vi "HK Channel Read Formatted Value.vi"(8 "error in (no error)":errorcluster, 10 "Name":string, 11 "HK Channel in":refnum<class "HK Table.lvclass">) -> (0 "error out":errorcluster, 1 "Units":string, 2 "Value Formatted":string, 3 "HK Channel out":refnum<class "HK Table.lvclass">, 4 "Avg. Formatted":string)   [LabVIEW 2019, in "HK Table.lvclass"]
uses:
  HK Table.lvclass
  HK Table.lvclass/HK Table.ctl
  HK Item/HK Item.lvclass/HK Item.ctl
  HK Item/HK Item.lvclass
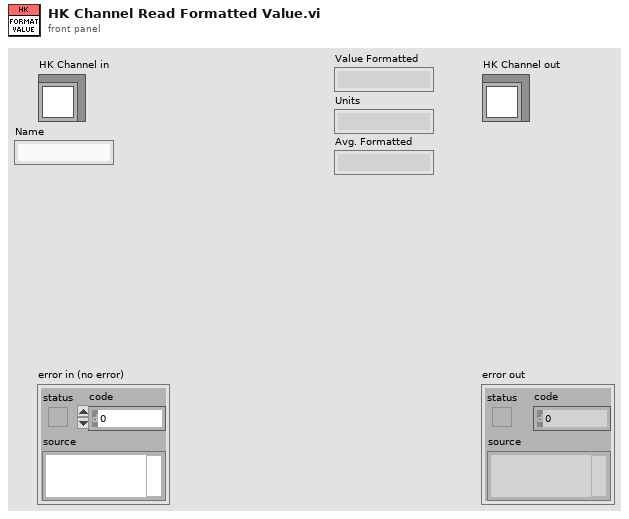
[diagram p1: front panel]
types:
  T1 = typedef "HK Item.lvclass/HK Channel Units and Setup.ctl" = cluster{"Unit Type":string, "Units":string, "Configuration":string, "Digits":i32, "Data Type":T2}
  T2 = typedef "HK Item.lvclass/HK Channel enum Data Type.ctl" = enum16{"Floating Point", "Integer", "Enum", "String", "Waveform", "File"}
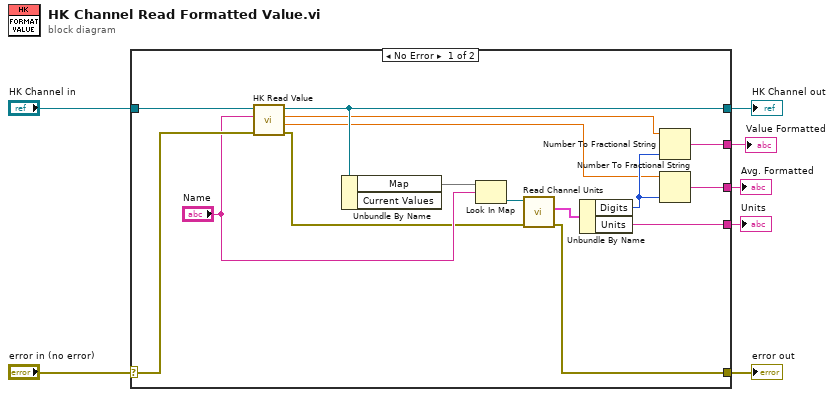
[diagram p0: block diagram]
diagram:
  n1 = case shown="No Error" "error in (no error)" {
    selector: "error in (no error)" -> [w19 w24]
    tunnel: [w12 w24] -> w6
    tunnel: [w21 w23] -> w4
    tunnel: "HK Channel in" -> [w20 w23]
    tunnel: [w15 _] -> w3
    tunnel: [w14 _] -> w1
    tunnel: [w8 _] -> w2
    frame No Error {
      n2 = call-dynamic "HK Read Value.vi"("error in (no error)"=w19, "Channel Name"="Name", "HK Channel in"=w20) -> ("error out"=w13:errorcluster, "Running Avg."=w9:dbl, "Value"=w11:dbl, "HK Channel out"=w21:refnum<class "HK Table.lvclass">)  [unwired: 3 in, 2 out]
      n3 = Unbundle By Name(w21) -> ("Map"=w22:map{string, refnum<class "HK Item.lvclass">})  [unwired: 1 out]
      n4 = Look In Map(map=w22, key="Name") -> (value=w17:refnum<class "HK Item.lvclass">)  [unwired: 1 in, 1 out]
      n5 = call "Read Channel Units.vi"("error in (no error)"=w13, "HK Item in"=w17) -> ("error out"=w12:errorcluster, "Channel Setup"=w16:T1)  [unwired: 7 in, 1 out]
      n6 = Unbundle By Name(w16) -> ("Digits"=w10:i32, "Units"=w15:string)
      n7 = Number To Fractional String(number=w11, precision (6)=w10) -> (F-format string=w8:string)  [unwired: 2 in]
      n8 = Number To Fractional String(number=w9, precision (6)=w10) -> (F-format string=w14:string)  [unwired: 2 in]
    }
    frame Error {
    }
  }
  "error out" <- w6
  "HK Channel out" <- w4
  "Value Formatted" <- w2
  "Units" <- w3
  "Avg. Formatted" <- w1
